vi "FTW-Event-Deserialize-JSON.vi"(0 "Serialized Event":string, 11 "error in":errorcluster) -> (4 "Event":T1 {"Timestamp" format="%<%Y-%m-%d %H:%M:%S%03u>T"; "Uptime" format="%.3ps"}, 15 "error out":errorcluster)   [LabVIEW 2018]
uses:
  FTW-Event.ctl
  510915fe-9f74-482d-9897-7b3a07fe775f.vi
  JSON/core/FTW-JSON-Core-EncodingFlags.vi
  Reflection/FTW-Reflection-Type.vi
  JSON/FTW-JSON-Parse.vi
  container/FTW-Container-GetFlattenedValue.vi
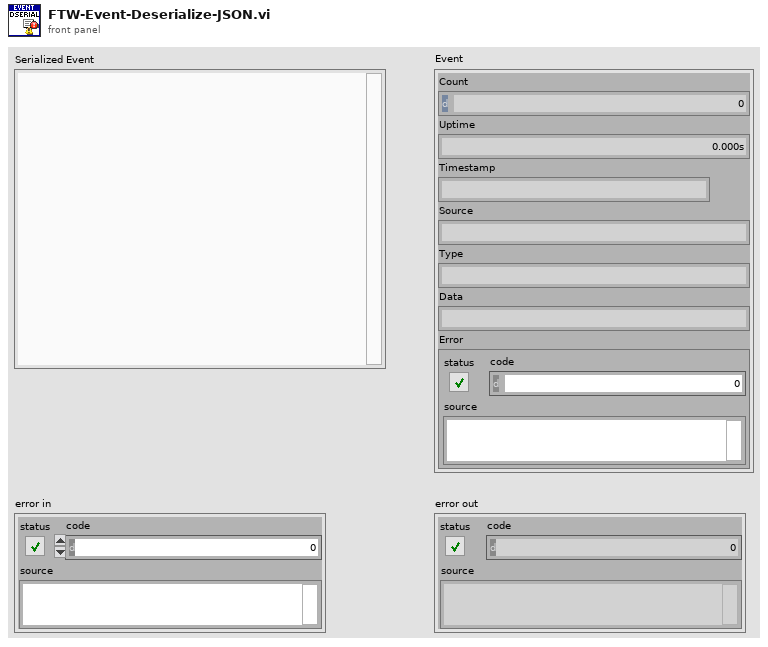
[diagram p1: front panel]
types:
  T1 = typedef "FTW-Event.ctl" = cluster{"Count":i32, "Uptime":dbl, "Timestamp":timestamp, "Source":string, "Type":string, "Data":string, "Error":errorcluster}
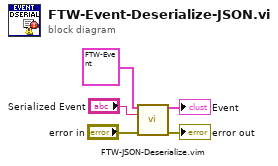
[diagram p0: block diagram]
diagram:
  n1 = call "FTW-JSON-Deserialize.vim"("Type In"=T1 {"Count"=0, "Uptime"=0.0, "Timestamp"=timestamp(0 s since 1904-01-01), "Source"="", "Type"="", "Data"="", "Error"={"status"=FALSE, "code"=0, "source"=""}} ("Event"), "JSON String"="Serialized Event", "error in"="error in") -> ("Type Out"=→"Event":T1, "error out"=→"error out":errorcluster)  [unwired: 11 in]
